vi "u2pwm.vi"(2 "error in (no error)":errorcluster, 3 "u":dbl) -> (0 "error out":errorcluster, 1 "PWM":dbl)   [LabVIEW 2019]
panel:
  out "fpwm":dbl
  out "b":dbl
  out "a":dbl
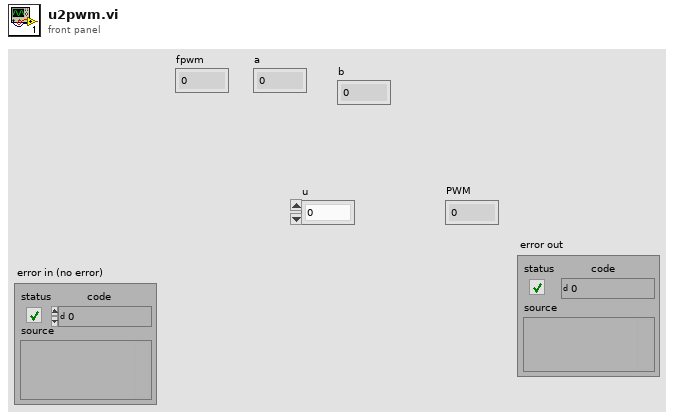
[diagram p1: front panel]
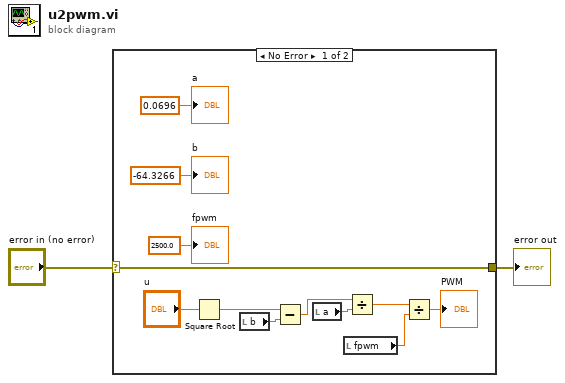
[diagram p0: block diagram]
diagram:
  n1 = case shown="No Error" "error in (no error)" {
    selector: "error in (no error)" -> [w3 w15]
    tunnel: [w3 w15] -> w1
    frame No Error {
      n2 = Square Root(x="u") -> (sqrt(x)=w10:dbl)
      n3 = local read "b"() -> (w9:dbl)
      n4 = Subtract(x=w10, y=w9) -> (x-y=w8:dbl)
      n5 = local read "a"() -> (w7:dbl)
      n6 = local read "fpwm"() -> (w4:dbl)
      n7 = Divide(x=w8, y=w7) -> (x/y=w6:dbl)
      n8 = Divide(x=w6, y=w4) -> (x/y=→"PWM":dbl)
      "a" <- 0.0696 ("a")
      "b" <- -64.3266 ("b")
      "fpwm" <- 2500.0 ("fpwm")
    }
    frame Error {
    }
  }
  "error out" <- w1
